vi "Coulomb's Law(SubVI).vi"(9 "r":dbl, 10 "q2":dbl, 11 "q1":dbl) -> (3 "F":dbl)   [LabVIEW 2024]
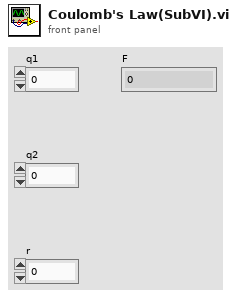
[diagram p1: front panel]
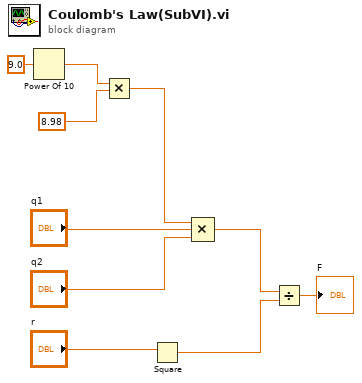
[diagram p0: block diagram]
diagram:
  n1 = Power Of 10(x=9.0) -> (10^x=w2:dbl)
  n2 = Multiply(x=w2, y=8.98) -> (x*y=w4:dbl)
  n3 = Square(x="r") -> (x^2=w9:dbl)
  n4 = Compound Arithmetic op=MULTIPLY(w4, "q1", "q2") -> (w8:dbl)
  n5 = Divide(x=w8, y=w9) -> (x/y=→"F":dbl)
